vi "Send CW to Radio.vi"(6 "Word Gap":u8, 7 "Character Gap":u8, 8 "error in":errorcluster, 9 "Unit Speed (sec)":dbl, 10 "Plaintext Array":string[](array[string]), 11 "Plaintext to CW Map":map{string, bool[]}(c390)) -> (0 "error out":errorcluster)   [LabVIEW 2026]
uses:
  125424c6-6355-497d-a8e3-58349ff11fee.vi
  8e32e904-5aaf-4f87-984d-a0d2a0ccfe3d.vi
  c1495b64-da55-4246-bd88-6f995fe51ef8.vi
  Libraries/FT-818 CW Key Control/FT-818 CW Key Control.lvlib
  b69b3da0-c846-40fb-a8af-64708a782255.vi
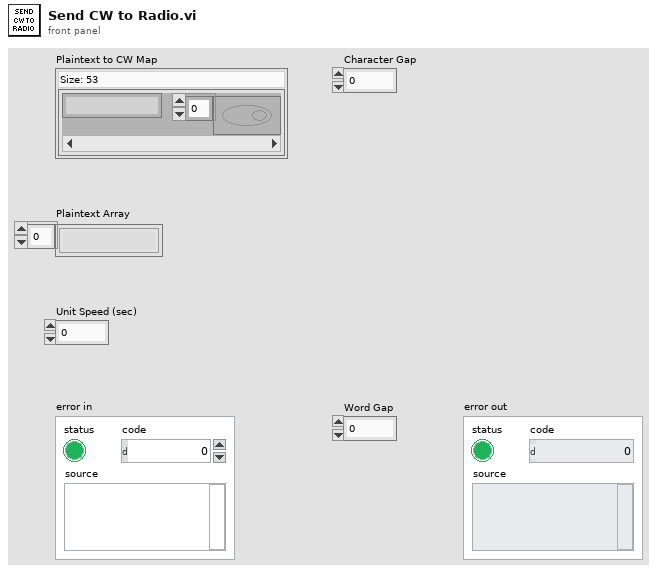
[diagram p1: front panel]
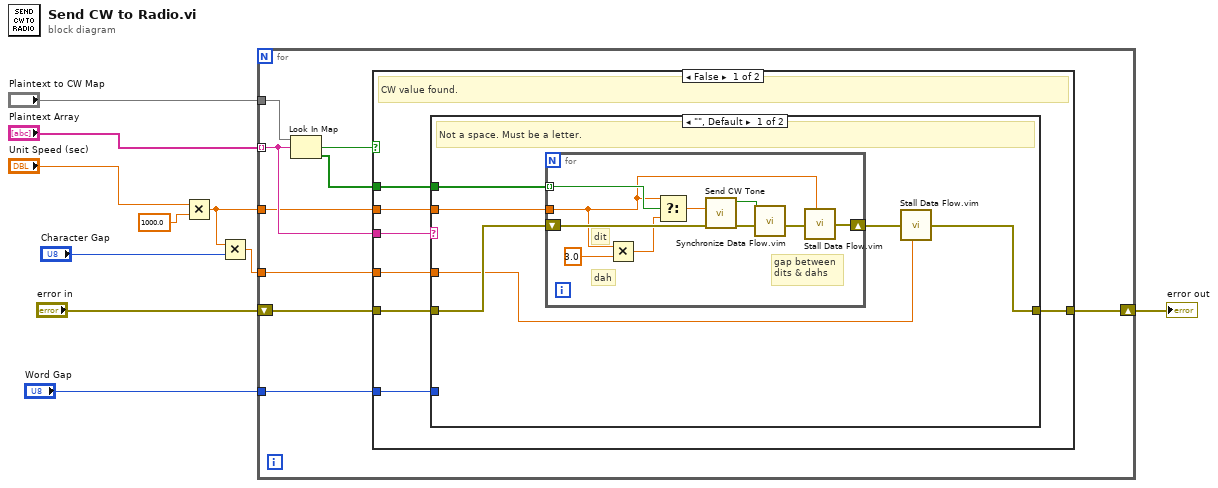
[diagram p0: block diagram]
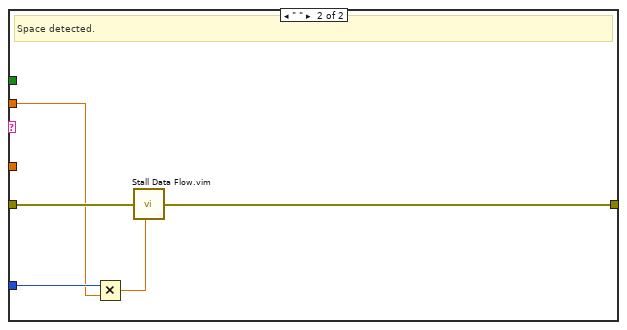
[diagram p2: hidden frame]
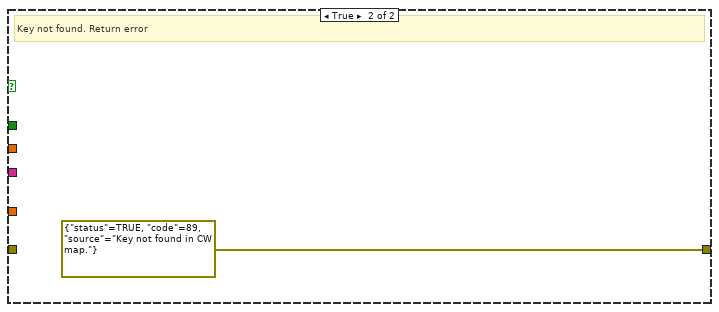
[diagram p3: hidden frame]
diagram:
  n1 = Multiply(x="Unit Speed (sec)", y=1000.0) -> (x*y=w3:dbl)
  n2 = Multiply(x=w3, y="Character Gap") -> (x*y=w1:dbl)
  n3 = for {
    tunnel: "Plaintext Array" -> [w15] mode=indexing
    tunnel: w3 -> [w14]
    tunnel: w1 -> [w12]
    tunnel: "Word Gap" -> [w11]
    shift-right: [w17] -> w8
    shift-left: "error in" -> [w13]
    tunnel: "Plaintext to CW Map" -> [w19]
    n4 = Look In Map(map=w19, key=w15) -> (key not found?=w18:bool, value=w16:bool[])  [unwired: 1 in]
    n5 = case shown="False" w18 {
      tunnel: [w21 errorcluster {"status"=TRUE, "code"=89, "source"="Key not found in CW map."} ("error out")] -> w17
      tunnel: w16 -> [w23 _]
      tunnel: w15 -> [w26 _]
      tunnel: w14 -> [w25 _]
      tunnel: w13 -> [w24 _]
      tunnel: w12 -> [w22 _]
      tunnel: w11 -> [w20 _]
      frame False {
        # "CW value found."
        n6 = case shown="\"\", Default" w26 {
          tunnel: w25 -> [w28 w43]
          tunnel: w24 -> [w32 w47]
          tunnel: w23 -> [w31 _]
          tunnel: w22 -> [w27 _]
          tunnel: [w29 w46] -> w21
          tunnel: w20 -> [_ w45]
          frame "", Default {
            # "Not a space. Must be a letter."
            n7 = for {
              shift-right: [w36] -> w30
              shift-left: w32 -> [w40]
              tunnel: w31 -> [w42] mode=indexing
              tunnel: w28 -> [w35]
              # "gap between\ndits & dahs"
              # "dit"
              # "dah"
              n8 = Multiply(x=w35, y=3.0) -> (x*y=w39:dbl)
              n9 = Select(t=w35, s=w42, f=w39) -> (s? t:f=w41:dbl)
              n10 = call "Send CW Tone.vi"("error in"=w40, "CW Tone Time (ms)"=w41) -> ("error out"=w37:errorcluster, "Done?"=w33:bool)  [unwired: 7 in, 1 out]
              n11 = call "Synchronize Data Flow.vim"("input 3"=w37, "input 1"=w33) -> ("output 3"=w34:errorcluster)  [unwired: 2 in, 3 out]
              n12 = call "Stall Data Flow.vim"("value in"=w34, "milliseconds to wait"=w35) -> ("value out"=w36:errorcluster)  [unwired: 1 out]
            }
            n13 = call "Stall Data Flow.vim"("value in"=w30, "milliseconds to wait"=w27) -> ("value out"=w29:errorcluster)  [unwired: 1 out]
          }
          frame " " {
            # "Space detected."
            n14 = Multiply(x=w45, y=w43) -> (x*y=w44:dbl)
            n15 = call "Stall Data Flow.vim"("value in"=w47, "milliseconds to wait"=w44) -> ("value out"=w46:errorcluster)  [unwired: 1 out]
          }
        }
      }
      frame True {
        # "Key not found. Return error"
      }
    }
  }
  "error out" <- w8
